vi "adaptWhiteBalance.vi"(0 "Camera in":refnum<class "Camera.lvclass">, 5 "data_format":T1(ring)=enum."Mono16", 7 "raw_image (U16)":u16[][](array[numeric]), 9 "roi":cluster{"x0":u64, "y0":u64, "x1":u64, "y1":u64}={"x0"=18446744073709551615, "y0"=18446744073709551615, "x1"=18446744073709551615, "y1"=18446744073709551615}, 11 "error in (no error)":errorcluster) -> (4 "Camera out":refnum<class "Camera.lvclass">, 15 "error out":errorcluster)   [LabVIEW 2019, in "Camera.lvclass"]
doc: "Get an image from the recorder. The type of the image is 2D array of pixel values. This array is\nshaped depending on the resolution and ROI of the image."
uses:
  Camera.lvclass
  pco.convert/Convert.lvlib
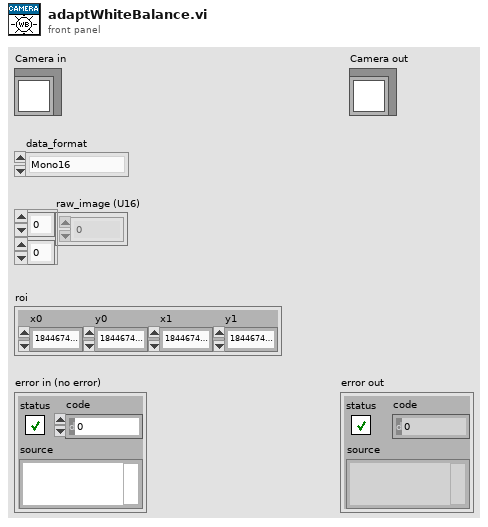
[diagram p1: front panel]
types:
  T1 = enum16{"Undefined", "Mono8", "Mono16", "BGRA8", "RGBA8", "BGRA16", "RGBA16", "CompressedMono8"}
  T2 = map{enum16{"Undefined", "Mono8", "Mono16", "BGRA8", "RGBA8", "BGRA16", "RGBA16", "CompressedMono8"}, cluster{"sharpen":bool, "adaptive_sharpen":bool, "flip_vertical":bool, "auto_minmax":bool, "min_limit":u16, "max_limit":u16, "gamma":dbl, "contrast":i32, "pco_debayer_algorithm":bool, "color_temperature":i32, "color_saturation":i32, "color_vibrance":i32, "color_tint":i32, "lut_file":path}}
  T3 = cluster{"sharpen":bool, "adaptive_sharpen":bool, "flip_vertical":bool, "auto_minmax":bool, "min_limit":u16, "max_limit":u16, "gamma":dbl, "contrast":i32, "pco_debayer_algorithm":bool, "color_temperature":i32, "color_saturation":i32, "color_vibrance":i32, "color_tint":i32, "lut_file":path}
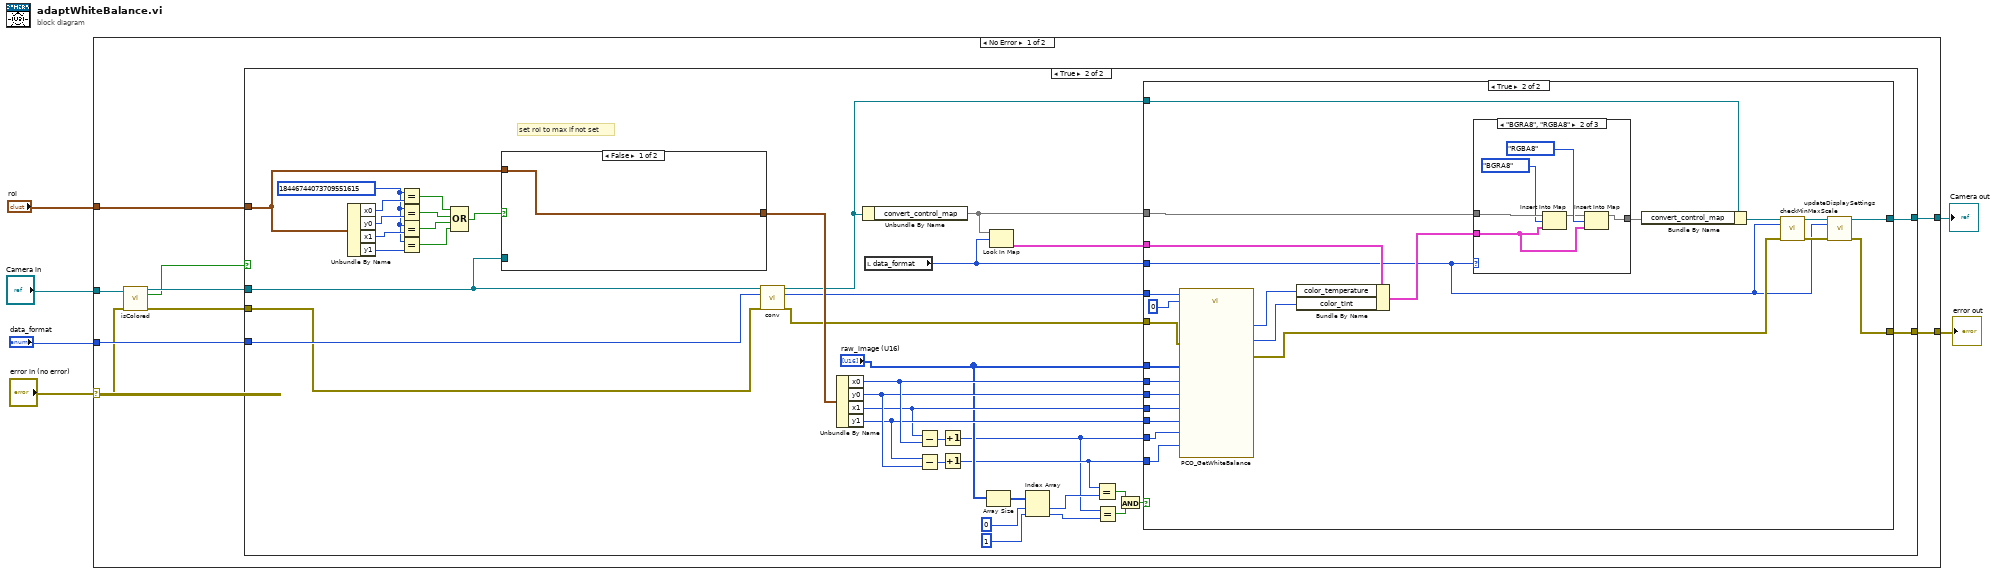
[diagram p0: block diagram]
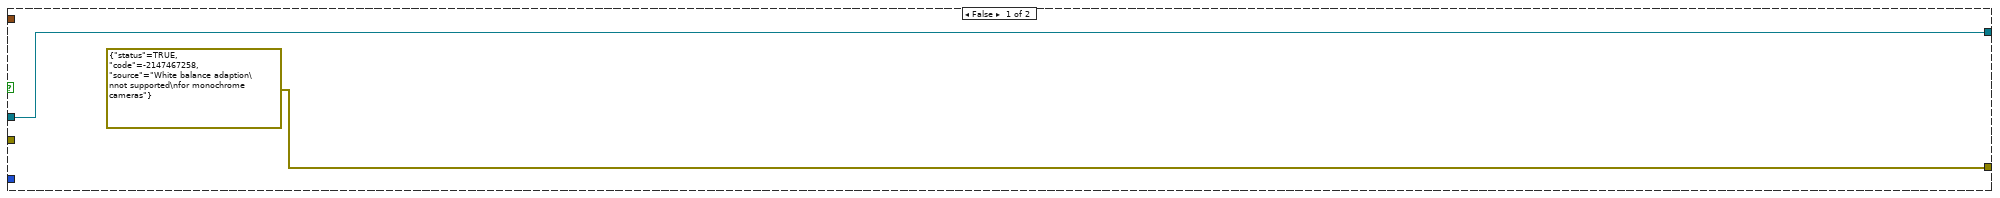
[diagram p2: hidden frame]
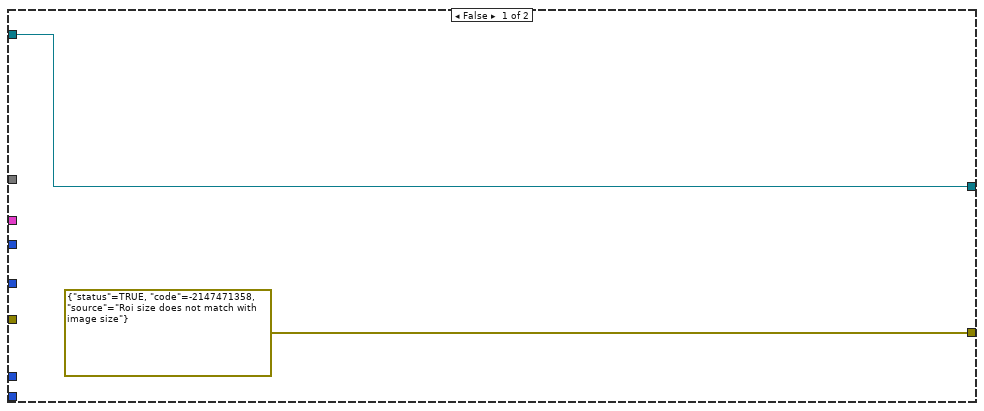
[diagram p3: hidden frame]
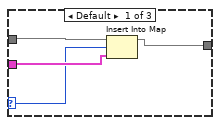
[diagram p4: hidden frame]
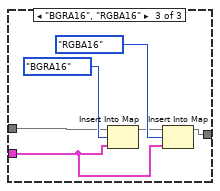
[diagram p5: hidden frame]
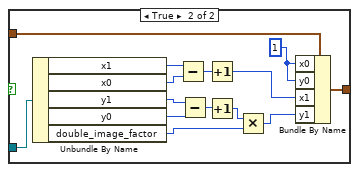
[diagram p6: hidden frame]
diagram:
  n1 = case shown="No Error" "error in (no error)" {
    selector: "error in (no error)" -> [w10 w115]
    tunnel: "Camera in" -> [w11 w116]
    tunnel: "roi" -> [w15 _]
    tunnel: "data_format" -> [w14 _]
    tunnel: [w13 w115] -> w2
    tunnel: [w12 w116] -> w1
    frame No Error {
      n2 = call-dynamic "isColored.vi"("Camera in"=w11, "error in (no error)"=w10) -> ("Camera out"=w9:refnum<class "Camera.lvclass">, "colored"=w7:bool, "error out"=w8:errorcluster)  [unwired: 11 in]
      n3 = case shown="True" w7 {
        tunnel: w15 -> [_ w47]
        tunnel: w14 -> [_ w46]
        tunnel: [errorcluster {"status"=TRUE, "code"=-2147467258, "source"="White balance adaption\nnot supported\nfor monochrome cameras"} ("error constant") w36] -> w13
        tunnel: [w16 w18] -> w12
        tunnel: w9 -> [w16 w24]
        tunnel: w8 -> [_ w23]
        frame False {
        }
        frame True {
          w49 = u64 18446744073709551615 ("x0")
          # "set roi to max if not set"
          n4 = Unbundle By Name(w47) -> ("x0"=w53:u64, "y0"=w52:u64, "x1"=w51:u64, "y1"=w50:u64)
          n5 = Equal?(x=w49, y=w53) -> (x = y?=w54:bool)
          n6 = Equal?(x=w49, y=w52) -> (x = y?=w55:bool)
          n7 = Equal?(x=w49, y=w51) -> (x = y?=w56:bool)
          n8 = Equal?(x=w49, y=w50) -> (x = y?=w57:bool)
          n9 = Compound Arithmetic op=OR(w54, w55, w56, w57) -> (w48:bool)
          n10 = case shown="False" w48 {
            tunnel: w24 -> [_ w114]
            tunnel: w47 -> [w100 w113]
            tunnel: [w100 w112] -> w45
            frame False {
            }
            frame True {
              w111 = u16 1 ("x0")
              n11 = Unbundle By Name(w114) -> ("x1"=w110:u64, "x0"=w109:u64, "y1"=w107:u64, "y0"=w106:u64, "double_image_factor"=w102:u16)
              n12 = Subtract(x=w110, y=w109) -> (x-y=w108:u64)
              n13 = Subtract(x=w107, y=w106) -> (x-y=w104:u64)
              n14 = Increment(x=w108) -> (x+1=w105:u64)
              n15 = Increment(x=w104) -> (x+1=w103:u64)
              n16 = Multiply(x=w103, y=w102) -> (x*y=w101:u64)
              n17 = Bundle By Name(cluster=w113, "x0"=w111, "y0"=w111, "x1"=w105, "y1"=w101) -> (w112:cluster{"x0":u64, "y0":u64, "x1":u64, "y1":u64})
            }
          }
          n18 = call-dynamic "conv.vi"("Camera in"=w24, "data_format"=w46, "error in (no error)"=w23) -> ("Camera out"=w22:refnum<class "Camera.lvclass">, "conv"=w37:u64, "error out"=w44:errorcluster)  [unwired: 10 in]
          n19 = Unbundle By Name(w45) -> ("x0"=w41:u64, "y0"=w40:u64, "x1"=w38:u64, "y1"=w39:u64)
          n20 = Unbundle By Name(w22) -> ("convert_control_map"=w21:T2)
          n21 = local read "data_format"() -> (w20:T1)
          n22 = Subtract(x=w38, y=w41) -> (x-y=w43:u64)
          n23 = Subtract(x=w39, y=w40) -> (x-y=w42:u64)
          n24 = Increment(x=w43) -> (x+1=w29:u64)
          n25 = Increment(x=w42) -> (x+1=w30:u64)
          n26 = Array Size(array="raw_image (U16)") -> (size(s)=w34:i32[])
          n27 = Look In Map(map=w21, key=w20) -> (value=w19:T3)  [unwired: 1 in, 1 out]
          n28 = Index Array(array=w34, index #1=0 ("index"), index #2=1 ("index")) -> (element #1=w31:i32, element #2=w28:i32)
          n29 = Equal?(x=w30, y=w31) -> (x = y?=w27:bool)
          n30 = Equal?(x=w29, y=w28) -> (x = y?=w26:bool)
          n31 = And(x=w27, y=w26) -> (x .and. y?=w25:bool)
          n32 = case shown="True" w25 {
            tunnel: w44 -> [_ w83]
            tunnel: w41 -> [_ w82]
            tunnel: w40 -> [_ w81]
            tunnel: w39 -> [_ w80]
            tunnel: w38 -> [_ w79]
            tunnel: w37 -> [_ w78]
            tunnel: [errorcluster {"status"=TRUE, "code"=-2147471358, "source"="Roi size does not match with image size"} ("error constant") w65] -> w36
            tunnel: "raw_image (U16)" -> [_ w74]
            tunnel: w30 -> [_ w76]
            tunnel: w29 -> [_ w75]
            tunnel: w22 -> [w58 w68]
            tunnel: w21 -> [_ w73]
            tunnel: w20 -> [_ w60]
            tunnel: w19 -> [_ w72]
            tunnel: [w58 w66] -> w18
            frame False {
            }
            frame True {
              n33 = call "PCO_GetWhiteBalance.vi"("ph"=w78, "mode"=0, "width"=w75, "height"=w76, "gb12"=w74, "x_min"=w82, "y_min"=w81, "error in (no error)"=w83, "x_max"=w79, "y_max"=w80) -> ("color_temp"=w71:i32, "tint"=w70:i32, "error out"=w62:errorcluster)  [unwired: 13 in, 2 out]
              n34 = Bundle By Name(cluster=w72, "color_temperature"=w71, "color_tint"=w70) -> (w69:T3)
              n35 = case shown="\"BGRA8\", \"RGBA8\"" w60 {
                selector: w60 -> [w85 _ _]
                tunnel: w73 -> [w86 w93 w95]
                tunnel: w69 -> [w87 w91 w94]
                tunnel: [w84 w88 w96] -> w67
                frame Default {
                  n36 = Insert Into Map(map in=w86, key=w85, value=w87) -> (map out=w84:T2)  [unwired: 2 out]
                }
                frame "BGRA8", "RGBA8" {
                  n37 = Insert Into Map(map in=w93, key=T1."BGRA8" ("data_format"), value=w91) -> (map out=w89:T2)  [unwired: 2 out]
                  n38 = Insert Into Map(map in=w89, key=T1."RGBA8" ("data_format"), value=w91) -> (map out=w88:T2)  [unwired: 2 out]
                }
                frame "BGRA16", "RGBA16" {
                  n39 = Insert Into Map(map in=w95, key=T1."BGRA16" ("data_format"), value=w94) -> (map out=w97:T2)  [unwired: 2 out]
                  n40 = Insert Into Map(map in=w97, key=T1."RGBA16" ("data_format"), value=w94) -> (map out=w96:T2)  [unwired: 2 out]
                }
              }
              n41 = Bundle By Name(cluster=w68, "convert_control_map"=w67) -> (w61:refnum<class "Camera.lvclass">)
              n42 = call-dynamic "checkMinMaxScale.vi"("Camera in"=w61, "data_format"=w60, "error in (no error)"=w62) -> ("Camera out"=w64:refnum<class "Camera.lvclass">, "error out"=w63:errorcluster)  [unwired: 10 in, 1 out]
              n43 = call-dynamic "updateDisplaySettings.vi"("Camera in"=w64, "data_format"=w60, "error in (no error)"=w63) -> ("Camera out"=w66:refnum<class "Camera.lvclass">, "error out"=w65:errorcluster)  [unwired: 11 in]
            }
          }
        }
      }
    }
    frame Error {
    }
  }
  "error out" <- w2
  "Camera out" <- w1
